vi "MLX Prog Init.vi"(7 "UseFastLIN":u8, 9 "BaudRateOfKbps":u8, 10 "LINChannel":u8, 11 "DeviceHandle":i32) -> (3 "function return":i32)   [LabVIEW 2010, in "mlx_programer.lvlib"]
doc: "int MLX_ProgInit(int DeviceHandle, unsigned char LINChannel,unsigned char BaudRateOfKbps,unsigned char UseFastLIN);"
uses:
  mlx_programer.lvlib
  USB2XXX/trunk/USB2XXX/USB2XXX/vs2010/Release/USB2XXX.dll
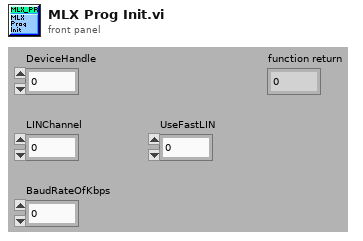
[diagram p1: front panel]
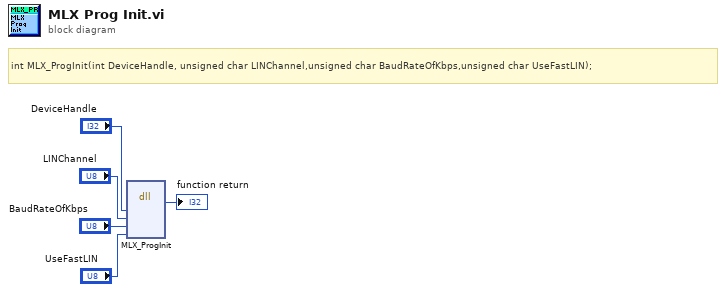
[diagram p0: block diagram]
diagram:
  # "int MLX_ProgInit(int DeviceHandle, unsigned char LINChannel,unsigned char BaudRateOfKbps,unsigned char UseFastLIN);"
  n1 = dll-call lib="E:/Projects/USB2XXX/trunk/USB2XXX/USB2XXX/vs2010/Release/USB2XXX.*" fn="MLX_ProgInit"("DeviceHandle"="DeviceHandle", "LINChannel"="LINChannel", "BaudRateOfKbps"="BaudRateOfKbps", "UseFastLIN"="UseFastLIN") -> (→"function return":i32)  [unwired: 7 in, 2 out]
